vi "sub vi - analog 1st setup v1.vi"() -> (1 "Graph 1":dynamicdata(graph), 2 "Graph 2":dynamicdata(graph), 3 "Graph 3":dynamicdata(graph), 4 "Error USB #0":bool, 6 "Error USB #1":bool, 8 "Error USB #2":bool, 10 "loop time":dbl format="%.6g")   [LabVIEW 2013]
panel:
  out "error out":errorcluster
  in  "Tab Control":enum32{"Page 1", "Page 2", "Page 3"}(tab)
  # "RUN THIS VERSION WITH ANALOG INPUT SET TO FALSE TO KICK START EXPRESS VI'S"
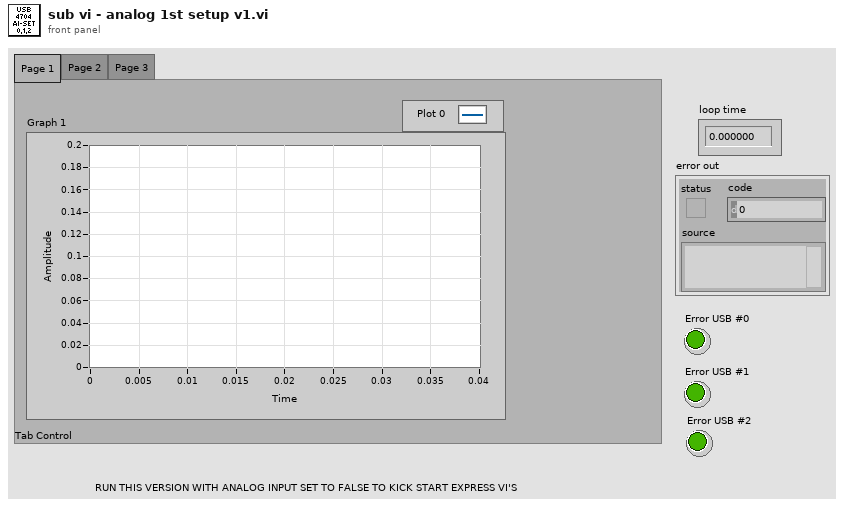
[diagram p1: front panel]
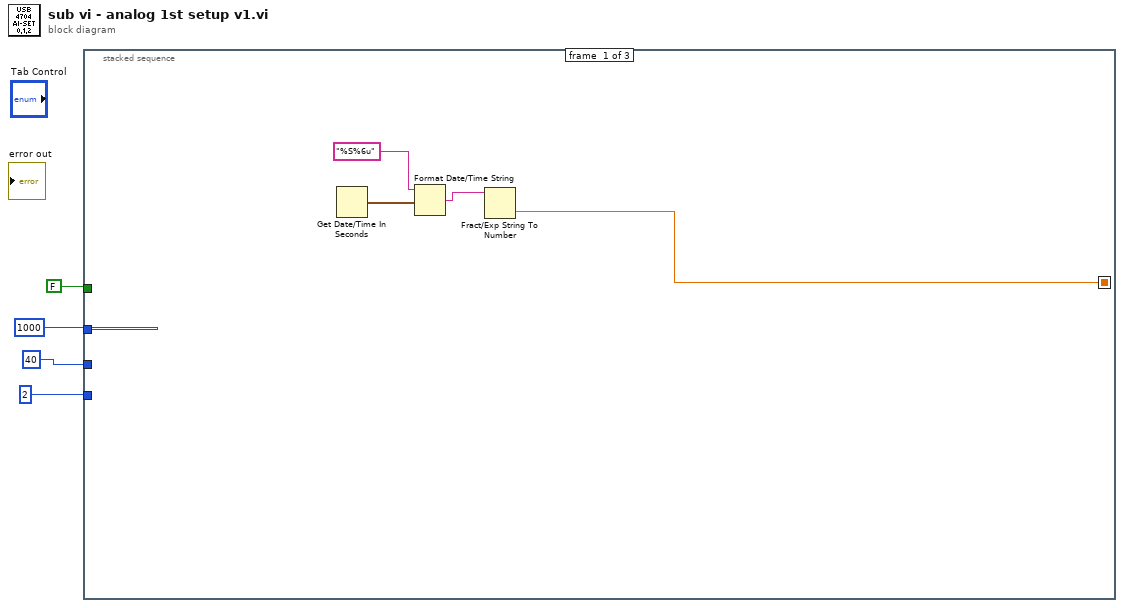
[diagram p0: block diagram]
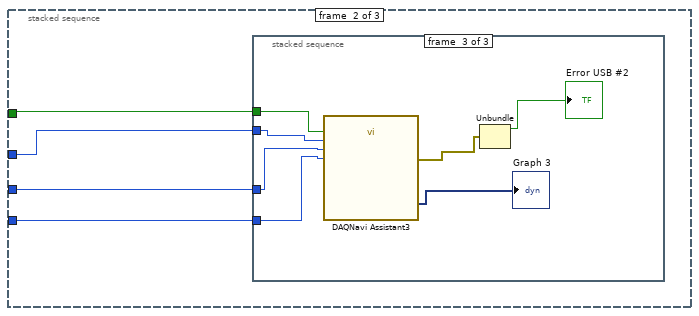
[diagram p2: hidden frame]
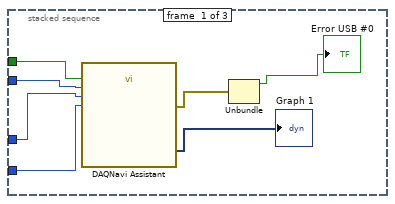
[diagram p3: hidden frame]
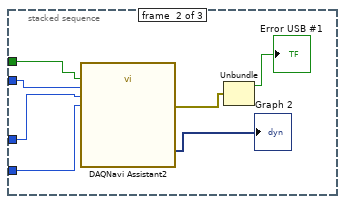
[diagram p4: hidden frame]
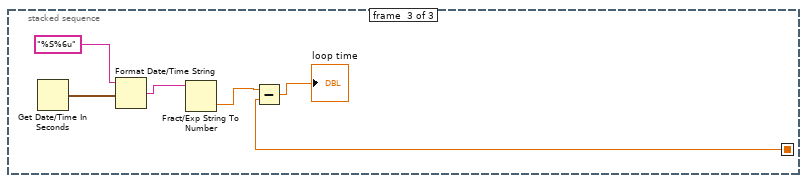
[diagram p5: hidden frame]
diagram:
  n1 = stacked-sequence {
    seq-local: [w5 _ _] -> [_ _ w35]
    tunnel: FALSE -> [_ w12 _]
    tunnel: 2 -> [_ w9 _]
    tunnel: 1000 -> [_ w11 _]
    tunnel: 40 -> [_ w10 _]
    frame #0 {
      n2 = Get Date/Time In Seconds() -> (seconds since 1Jan1904=w7:timestamp)
      n3 = Format Date/Time String(time format string (%c)="%S%6u", seconds (now)=w7) -> (date/time string=w6:string)  [unwired: 1 in]
      n4 = Fract/Exp String To Number(string=w6) -> (number=w5:dbl)  [unwired: 3 in, 1 out]
    }
    frame #1 {
      n5 = stacked-sequence {
        tunnel: w12 -> [w19 w26 w33]
        tunnel: w11 -> [w18 w25 w32]
        tunnel: w10 -> [w17 w24 w31]
        tunnel: w9 -> [w16 w23 w30]
        frame #0 {
          n6 = call "DAQNavi Assistant"("stop(true)"=w19, "conversion rate(Hz)"=w18, "samples"=w17, "time out(10s)"=w16) -> ("error out"=w14:errorcluster, "data out(DDT)"=→"Graph 1":dynamicdata)  [unwired: 22 in]
          n7 = Unbundle(w14) -> ("status"=→"Error USB #0":bool)  [unwired: 2 out]
        }
        frame #1 {
          n8 = call "DAQNavi Assistant2"("stop(true)"=w26, "conversion rate(Hz)"=w25, "samples"=w24, "time out(10s)"=w23) -> ("error out"=w22:errorcluster, "data out(DDT)"=→"Graph 2":dynamicdata)  [unwired: 22 in]
          n9 = Unbundle(w22) -> ("status"=→"Error USB #1":bool)  [unwired: 2 out]
        }
        frame #2 {
          n10 = call "DAQNavi Assistant3"("stop(true)"=w33, "conversion rate(Hz)"=w32, "samples"=w31, "time out(10s)"=w30) -> ("error out"=w29:errorcluster, "data out(DDT)"=→"Graph 3":dynamicdata)  [unwired: 22 in]
          n11 = Unbundle(w29) -> ("status"=→"Error USB #2":bool)  [unwired: 2 out]
        }
      }
    }
    frame #2 {
      n12 = Get Date/Time In Seconds() -> (seconds since 1Jan1904=w38:timestamp)
      n13 = Format Date/Time String(time format string (%c)="%S%6u", seconds (now)=w38) -> (date/time string=w37:string)  [unwired: 1 in]
      n14 = Fract/Exp String To Number(string=w37) -> (number=w36:dbl)  [unwired: 3 in, 1 out]
      n15 = Subtract(x=w36, y=w35) -> (x-y=→"loop time":dbl)
    }
  }
